vi "Refresh Palette.vi"(6 "Variant in":variant, 7 "Shift Pressed?":bool, 8 "error in (no error)":errorcluster, 10 "QD Combo Box Ref":refnum<vi>, 11 "QD Launch VI Ref":refnum<vi>) -> (0 "error out":errorcluster, 4 "Variant out":variant)   [LabVIEW 2017, in "Create a Place VI Contents.lvlib"]
doc: "After some change of the Control/Function palette, you can manually update the palette with this quickdrop."
uses:
  Create a Place VI Contents.lvlib
panel:
  in  "Undo Name":string="Refresh Pallette"
  # "Do not change the connector pane of this VI.\n\nSee the block diagram for directions on how to use this template."
  # "Specify the name of the Undo transaction"
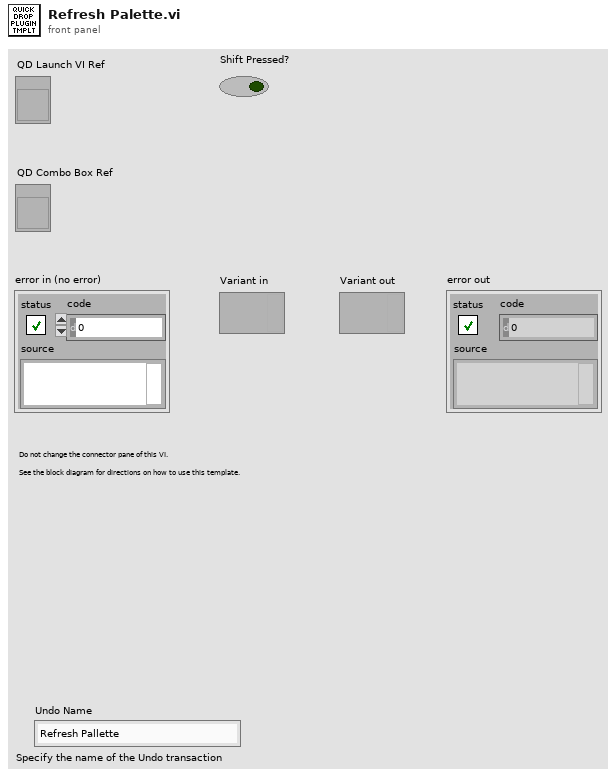
[diagram p1: front panel]
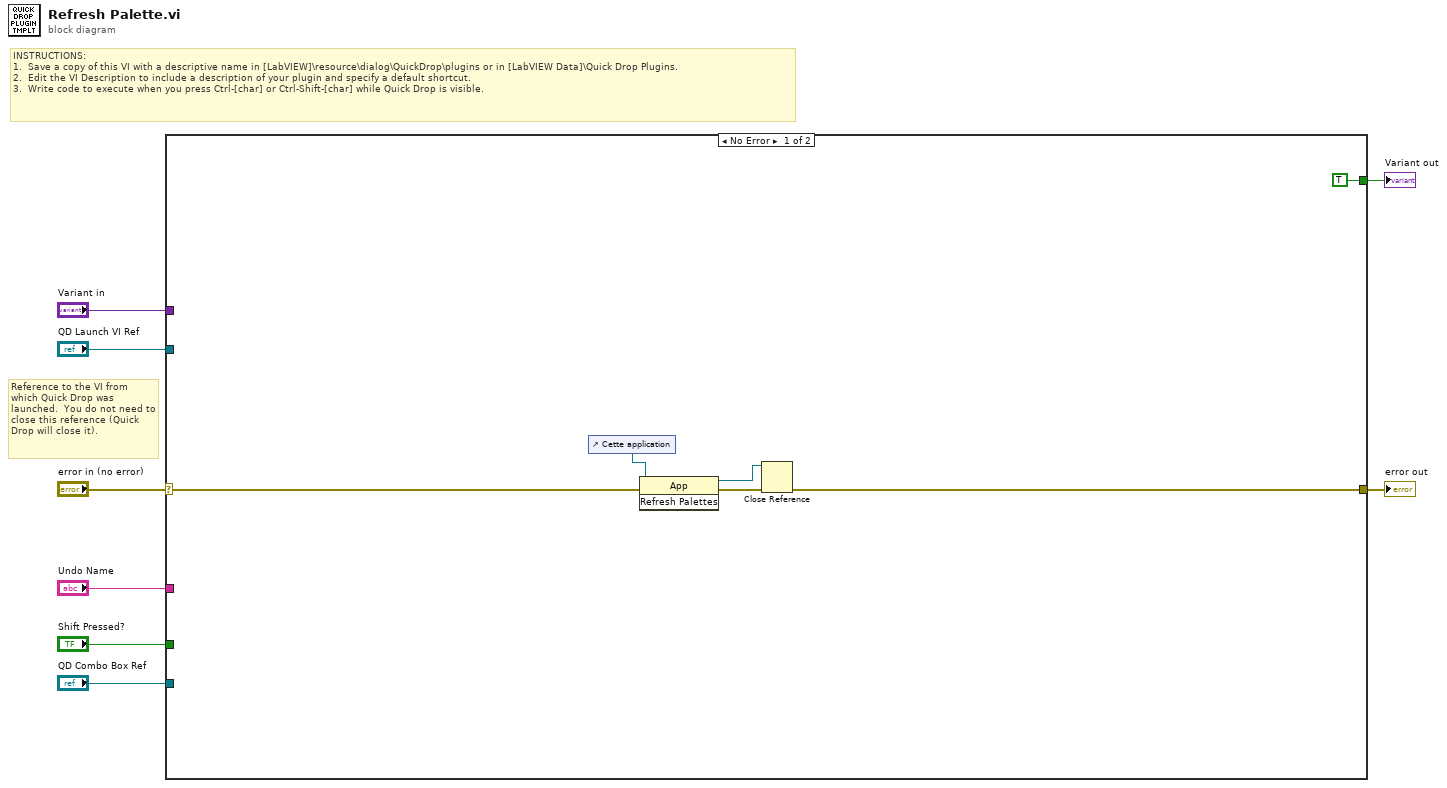
[diagram p0: block diagram]
diagram:
  # "Reference to the VI from which Quick Drop was launched.  You do not need to close this reference (Quick Drop will close it)."
  # "INSTRUCTIONS:\n1.  Save a copy of this VI with a descriptive name in [LabVIEW]\\resource\\dialog\\QuickDrop\\plugins or in [LabVIEW Data]\\Quick Drop Plugins.\n2.  Edit the VI Description to include a description of your plugin and specify a default shortcut. \n3.  Write code to execute when you press Ctrl-[char] or Ctrl-Shift-[char] while Quick Drop is visible."
  n1 = case shown="No Error" "error in (no error)" {
    selector: "error in (no error)" -> [w14 w15]
    tunnel: [w9 w15] -> w7
    tunnel: "QD Launch VI Ref" -> [_ _]
    tunnel: "Shift Pressed?" -> [_ _]
    tunnel: "QD Combo Box Ref" -> [_ _]
    tunnel: "Variant in" -> [_ _]
    tunnel: "Undo Name" -> [_ _]
    tunnel: [TRUE _] -> w1
    frame No Error {
      n2 = control-ref of="Cette application"() -> (w10:refnum<vi>)
      n3 = invoke class="App" method="Refresh Palettes"(reference=w10, error in=w14) -> (reference out=w11:refnum<vi>, error out=w12:errorcluster)  [unwired: 1 in, 1 out]
      n4 = Close Reference(reference=w11, error in (no error)=w12) -> (error out=w9:errorcluster)
    }
    frame Error {
    }
  }
  "error out" <- w7
  "Variant out" <- w1
